vi "Find Item in PPL.vi"(8 "error in (no error)":errorcluster, 9 "Target":refnum<vi>, 10 "default path":path, 11 "qualified name":string) -> (0 "error out":errorcluster, 1 "ppl exists?":bool, 2 "item path out":path)   [LabVIEW 2020, in "Message Maker.lvlib"]
uses:
  Message Maker.lvlib
  <vilib>/Utility/LVLibp/NI_PackedLibraryUtility.lvlib
  AFPP Shared/Constants.vi
  AFPP Shared/AFPP Shared.lvlib
  <resource>/dialog/lvconfig.llb/LV Config Read Pathlist.vi
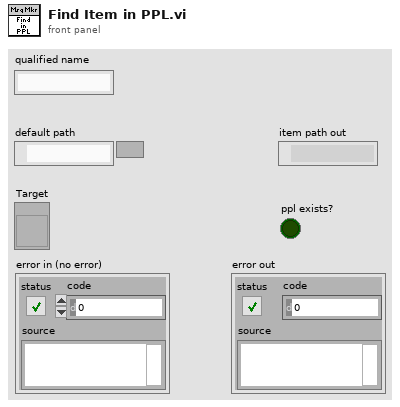
[diagram p1: front panel]
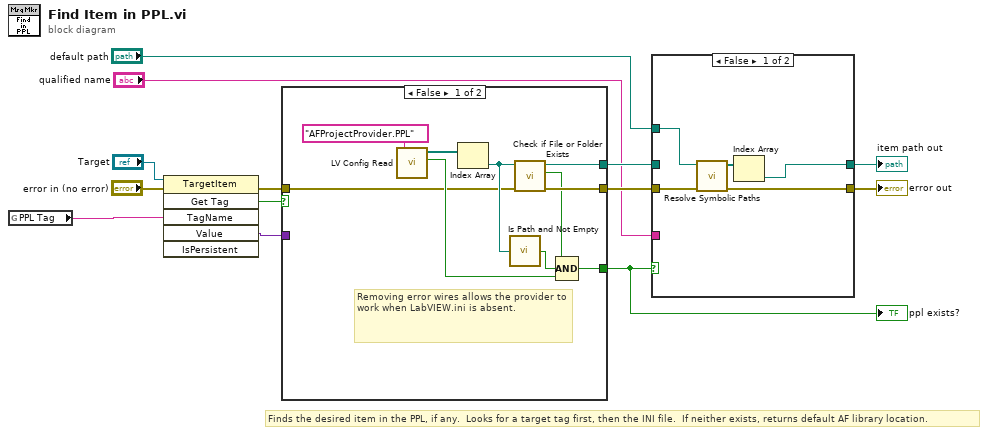
[diagram p0: block diagram]
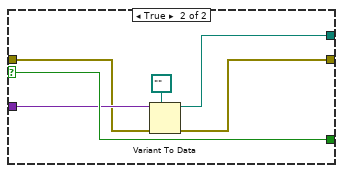
[diagram p2: hidden frame]
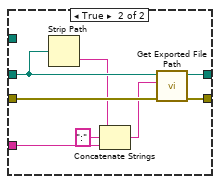
[diagram p3: hidden frame]
diagram:
  # "Finds the desired item in the PPL, if any.  Looks for a target tag first, then the INI file.  If neither exists, returns default AF library location."
  n1 = global read "Constants.vi" "PPL Tag"() -> (w1:string)
  n2 = invoke class="TargetItem" method="Get Tag"(reference="Target", error in="error in (no error)", "TagName"=w1) -> (error out=w5:errorcluster, "GetTag"=w4:bool, "Value"=w3:variant)  [unwired: 3 in, 3 out]
  n3 = case shown="False" w4 {
    selector: w4 -> [_ w29]
    tunnel: [w23 w24] -> w13
    tunnel: [w22 w26] -> w12
    tunnel: [w15 w29] -> w8
    tunnel: w5 -> [w14 w27]
    tunnel: w3 -> [_ w28]
    frame False {
      # "Removing error wires allows the provider to work when LabVIEW.ini is absent."
      n4 = call-poly <resource>:"LV Config Read.vi"("key"="AFProjectProvider.PPL") -> ("found?"=w18:bool, "value"=w21:path[])  [unwired: 4 in, 1 out]
      n5 = Index Array(array=w21) -> (element=w17:path)  [unwired: 1 in]
      n6 = call <vilib>:"Is Path and Not Empty.vi"("path"=w17) -> ("Is Path and Not Empty?"=w16:bool)  [unwired: 4 in]
      n7 = call <vilib>:"Check if File or Folder Exists.vi"("error in (no error)"=w14, "path"=w17) -> ("error out"=w22:errorcluster, "file or folder exists?"=w19:bool, "dup path"=w23:path)  [unwired: 7 in]
      n8 = Compound Arithmetic op=AND(w19, w16, w18) -> (w15:bool)
    }
    frame True {
      n9 = Variant To Data(error in=w27, type=path "", Variant=w28) -> (data=w24:path, error out=w26:errorcluster)
    }
  }
  "ppl exists?" <- w8
  n10 = case shown="False" w8 {
    tunnel: w12 -> [w31 w42]
    tunnel: [w30 w40] -> w9
    tunnel: "default path" -> [w33 _]
    tunnel: [w34 w41] -> w10
    tunnel: w13 -> [_ w38]
    tunnel: "qualified name" -> [_ w39]
    frame False {
      n11 = call "Resolve Symbolic Paths.vi"("error in (no error)"=w31, "Path"=w33) -> ("error out"=w30:errorcluster, "Resolved Paths"=w32:path[])  [unwired: 8 in]
      n12 = Index Array(array=w32) -> (element=w34:path)  [unwired: 1 in]
    }
    frame True {
      n13 = Strip Path(path=w38) -> (name=w36:string)  [unwired: 1 out]
      n14 = Concatenate Strings(w36, ":" ("string"), w39) -> (w37:string)
      n15 = call <vilib>:"Get Exported File Path.vi"("error in (no error)"=w42, "qualified name"=w37, "packed library path"=w38) -> ("error out"=w40:errorcluster, "path"=w41:path)  [unwired: 7 in]
    }
  }
  "item path out" <- w10
  "error out" <- w9
